vi "Settings Dialog.vi"(8 "error in (no error)":errorcluster, 11 "Settings in":T1={"Hardware Configuration"={"DAQmx Channel"="", "Sample Rate"=1000.0, "DAQmx Task"="", "ResetInterp"=FALSE, "GainConstants"=[], "FilterCoefficients"=[], "ChannelNames"=[], "ActiveChannels"=[], "Display Rate"=1000, "ResponseExtension"=TRUE}, "Logging Configuration"={"Log File Base Path"=path "", "Samples to Save"=0, "Trigger - Threshold"=0.0, "Trigger - Channel"=0, "Always Log"=FALSE, "External Trigger"=FALSE, "External Trigger Armed"=FALSE, "TDMS File Reference"=refnum, "DAQVersion"="", "SWVersion"="", "CircSamples"=0, "BeepWhenComplete"=FALSE, "ChannelConfig"=[], "ActiveChannels"=[], "Title"="", "Description"="", "ChannelNames"=[], "ResponseExtension"=TRUE}}) -> (0 "error out":errorcluster, 1 "Cancelled?":bool=TRUE, 2 "UI Refresh Needed?":bool, 3 "Settings out":T1={"Hardware Configuration"={"DAQmx Channel"="", "Sample Rate"=1000.0, "DAQmx Task"="", "ResetInterp"=FALSE, "GainConstants"=[], "FilterCoefficients"=[], "ChannelNames"=[], "ActiveChannels"=[], "Display Rate"=1000, "ResponseExtension"=TRUE}, "Logging Configuration"={"Log File Base Path"=path "C:/Users/jpassiak/Documents/LabVIEW Data/Logged Data.tdms", "Samples to Save"=0, "Trigger - Threshold"=0.0, "Trigger - Channel"=0, "Always Log"=FALSE, "External Trigger"=FALSE, "External Trigger Armed"=FALSE, "TDMS File Reference"=refnum, "DAQVersion"="", "SWVersion"="", "CircSamples"=0, "BeepWhenComplete"=FALSE, "ChannelConfig"=[], "ActiveChannels"=[], "Title"="", "Description"="", "ChannelNames"=[], "ResponseExtension"=TRUE}})   [LabVIEW 2017, in "Settings.lvlib"]
doc: "Dialog for selecting user specified settings."
uses:
  Settings.lvlib
  Settings.ctl
  Acquisition/Hardware Configuration.ctl
  Logging/Logging Configuration.ctl
  <vilib>/Utility/xml.llb/Write to XML File(string).vi
  Acquisition/Acquisition.lvlib
  Logging/Logging.lvlib
panel:
  in  "Tab Control 2":enum32{"Logging", "Channels", "Description"}(tab)=enum."Description"
  in  "Log File Path":path
  in  "Always Log":bool
  in  "Trigger Threshold\n [mm/s]":dbl min=0.0 max=100.0
  in  "Trigger Channel":u32(ring)=1 items=["CH1X", "CH1Y", "CH1Z"]
  in  "Channel Trigger":bool
  in  "Record Length [s]":u32=2
  in  "External Trigger":bool
  in  "Sample Rate [Hz]":u32=1000 min=4 max=1000
  in  "Pre-Trigger Buffer[s]":u32=2
  in  "Beep When Complete":bool=TRUE
  in  "Sensor response extension to 1Hz":bool=TRUE
  in  "Display Rate":i32=250 min=250 max=1000 step=10
  in  "Multicolumn Listbox":i32[](listbox)
  in  "Select Channels":i32[](listbox)
  in  "Description":string="..."
  in  "Title":string="Vibration Measurement"
  in  "Cancel Button":bool
  in  "OK Button":bool
  # "Non visible portion of dialog (needed for connector pane)."
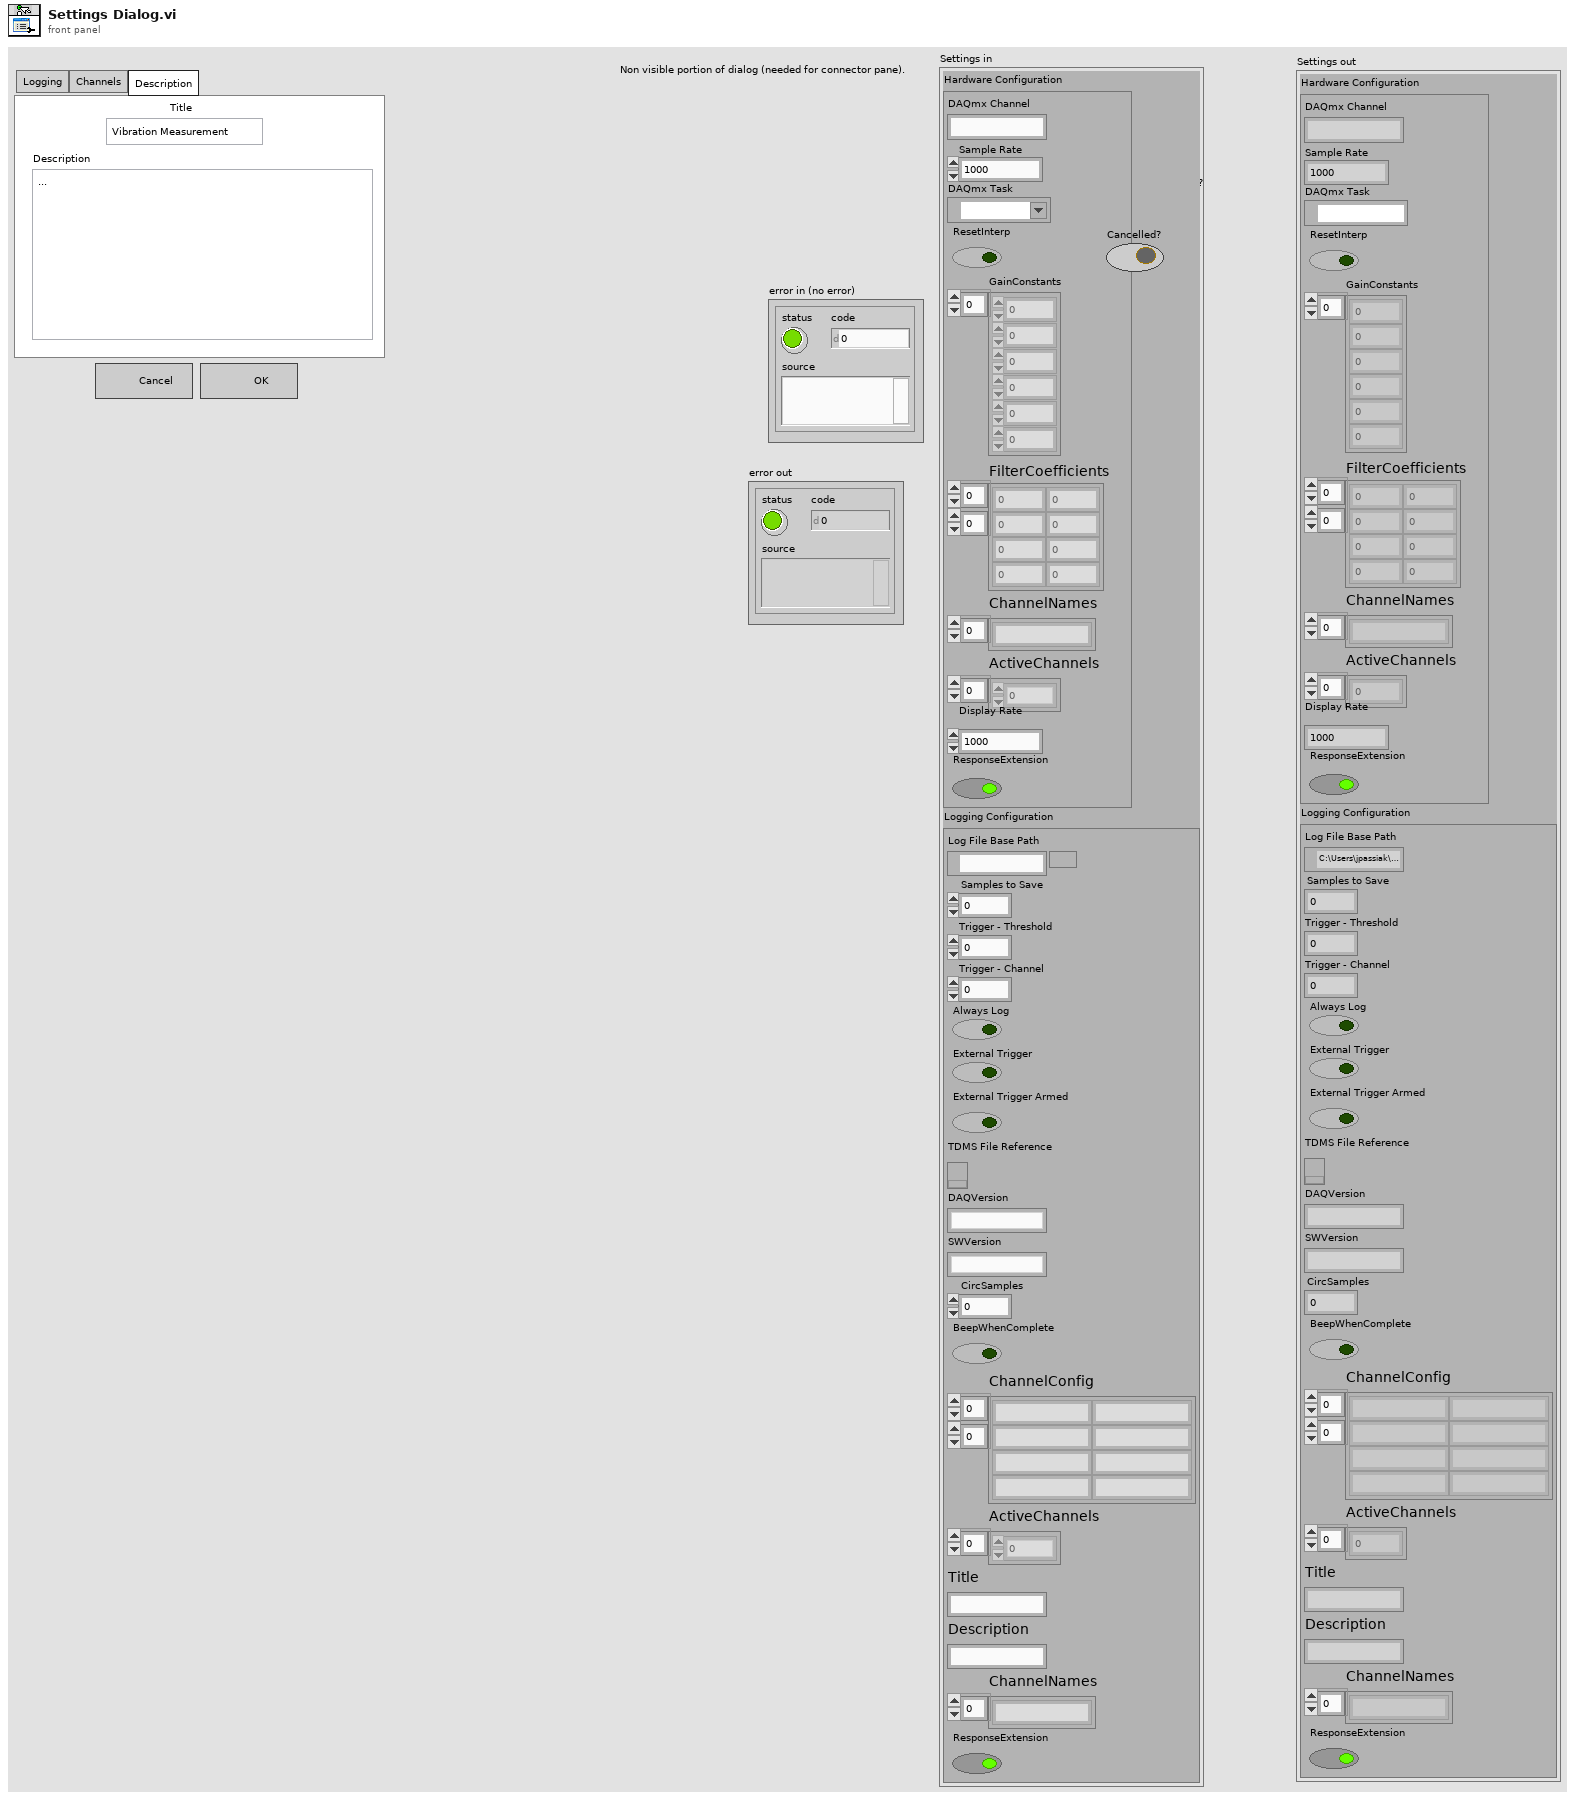
[diagram p1: front panel]
types:
  T1 = typedef "Settings.lvlib/Settings.ctl" = cluster{"Hardware Configuration":T2, "Logging Configuration":T3}
  T2 = typedef "Acquisition.lvlib/Hardware Configuration.ctl" = cluster{"DAQmx Channel":string, "Sample Rate":dbl, "DAQmx Task":refnum<k21>, "ResetInterp":bool, "GainConstants":dbl[], "FilterCoefficients":dbl[][], "ChannelNames":string[], "ActiveChannels":i32[], "Display Rate":i32, "ResponseExtension":bool}
  T3 = typedef "Logging.lvlib/Logging Configuration.ctl" = cluster{"Log File Base Path":path, "Samples to Save":u32, "Trigger - Threshold":dbl, "Trigger - Channel":u32, "Always Log":bool, "External Trigger":bool, "External Trigger Armed":bool, "TDMS File Reference":refnum<k34>, "DAQVersion":string, "SWVersion":string, "CircSamples":u32, "BeepWhenComplete":bool, "ChannelConfig":string[][], "ActiveChannels":i32[], "Title":string, "Description":string, "ChannelNames":string[], "ResponseExtension":bool}
  T4 = typedef "LVPoint32TypeDef.ctl" = cluster{"Horizontal":i32, "Vertical":i32}
  T5 = typedef "LVRowAndColumnTypeDef.ctl" = cluster{"Row":i32, "Column":i32}
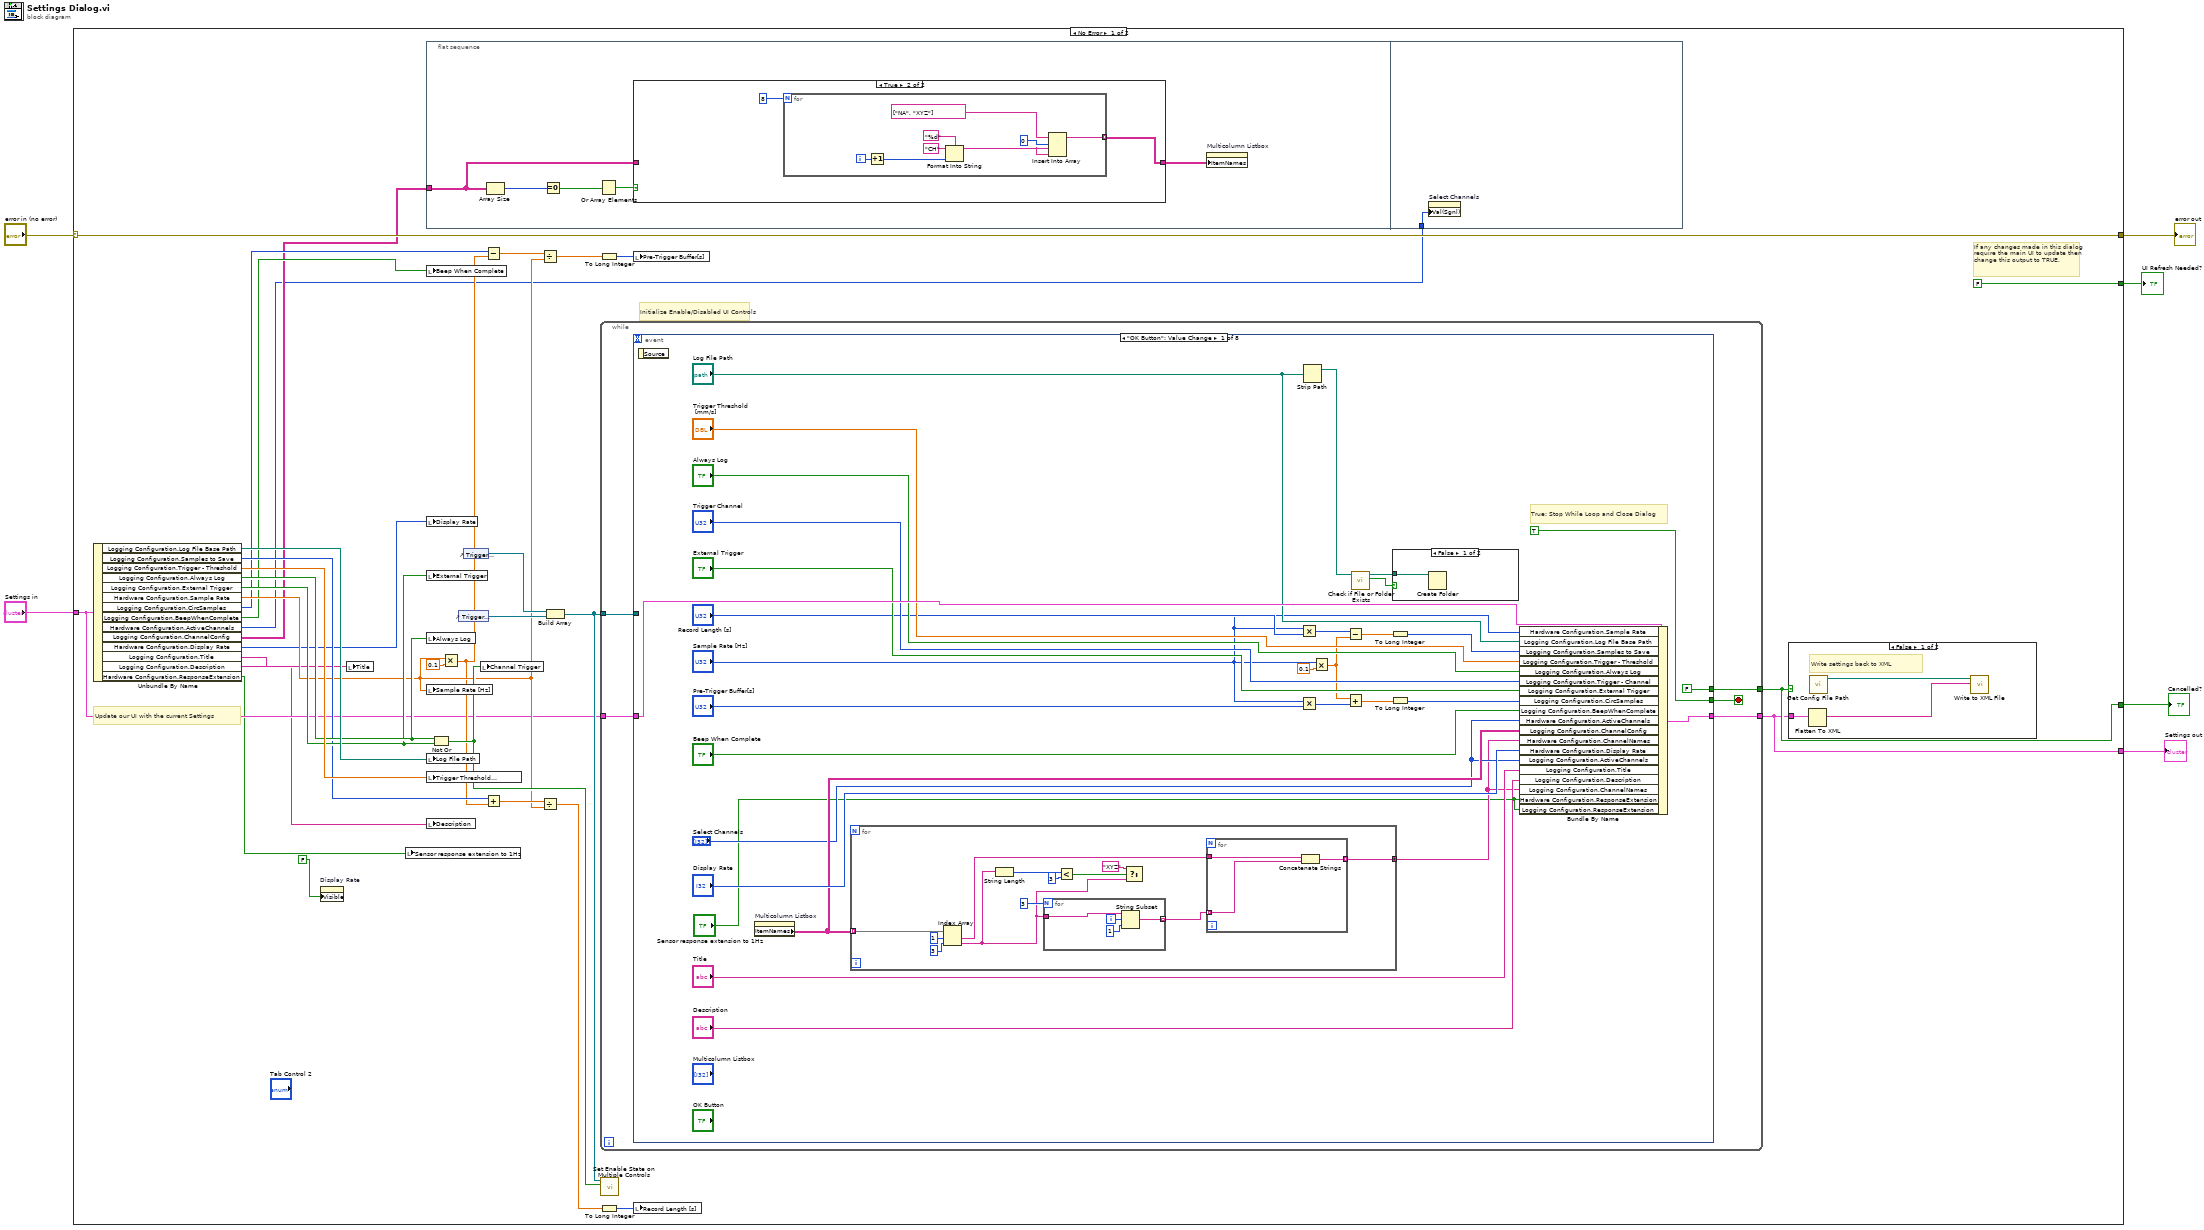
[diagram p0: block diagram]
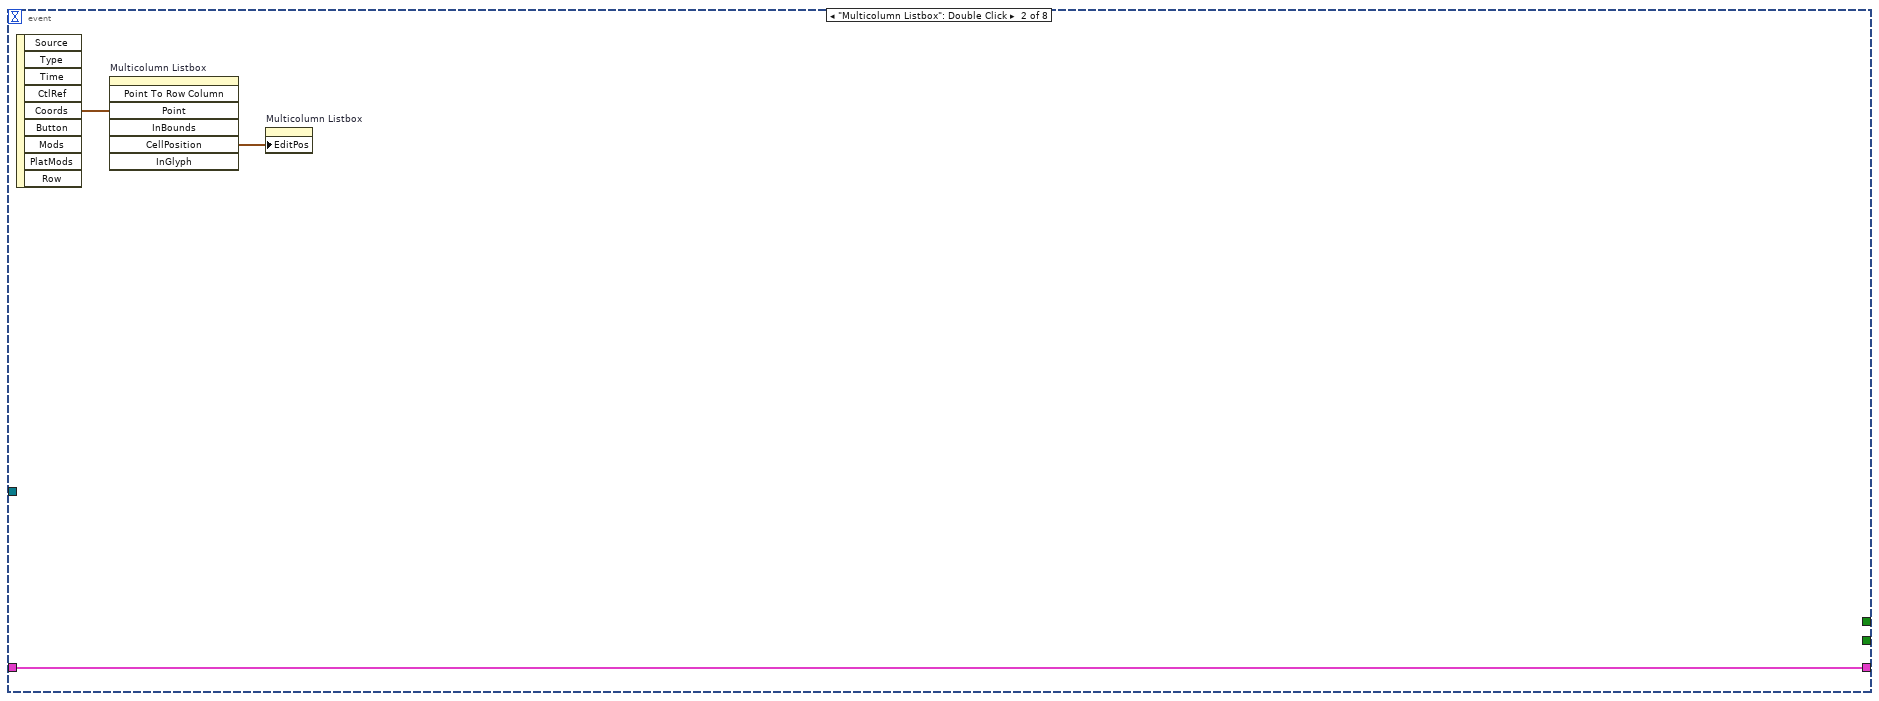
[diagram p4: hidden frame]
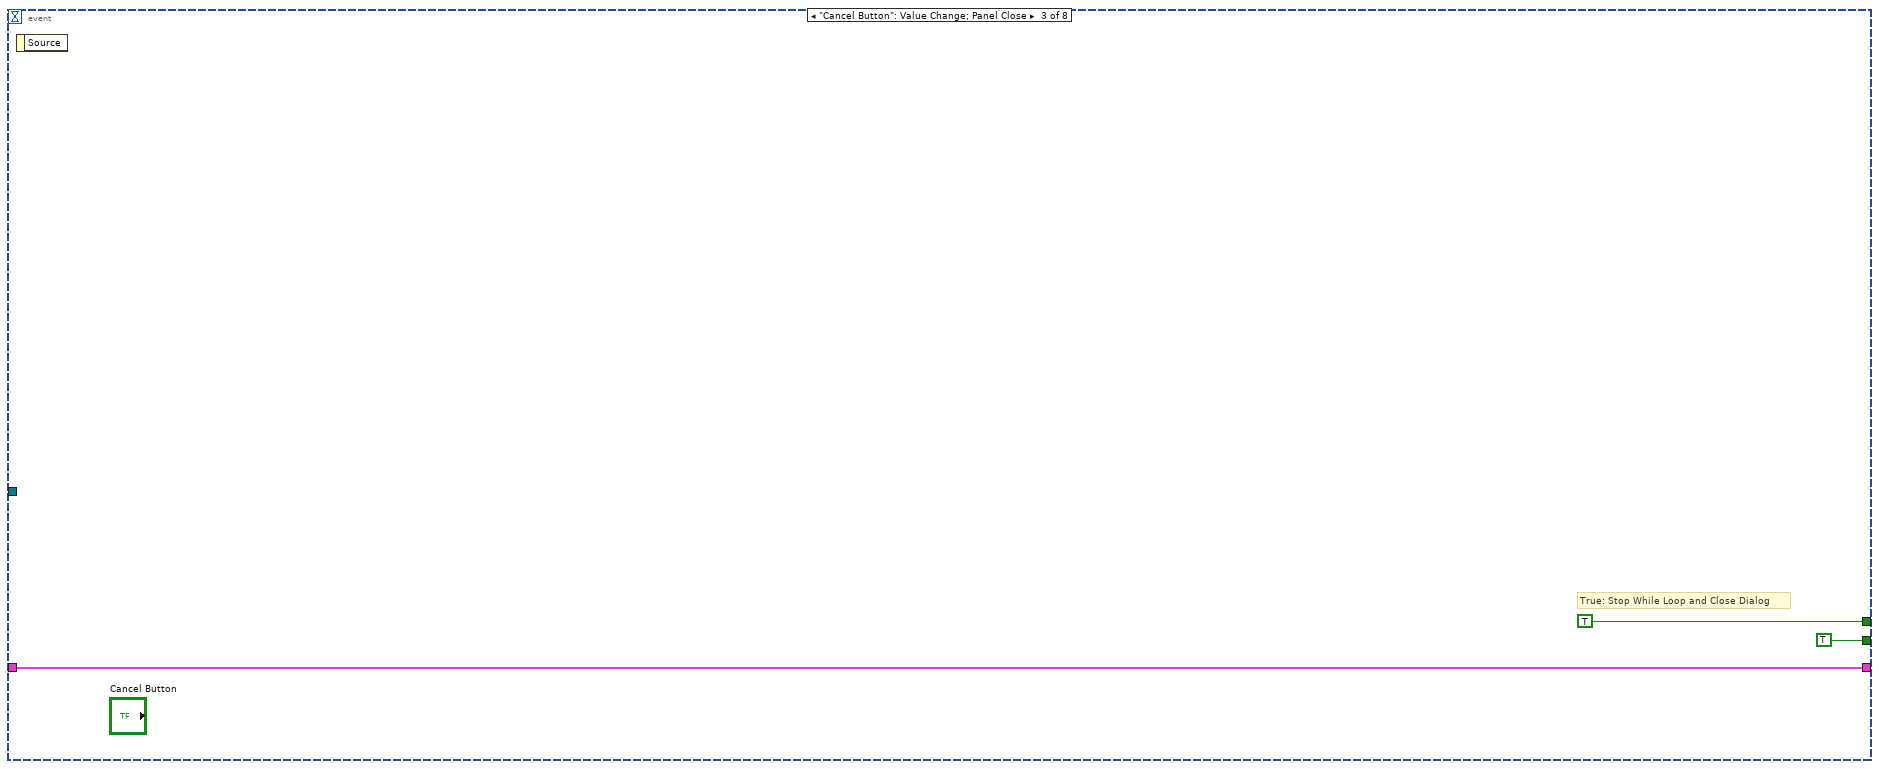
[diagram p5: hidden frame]
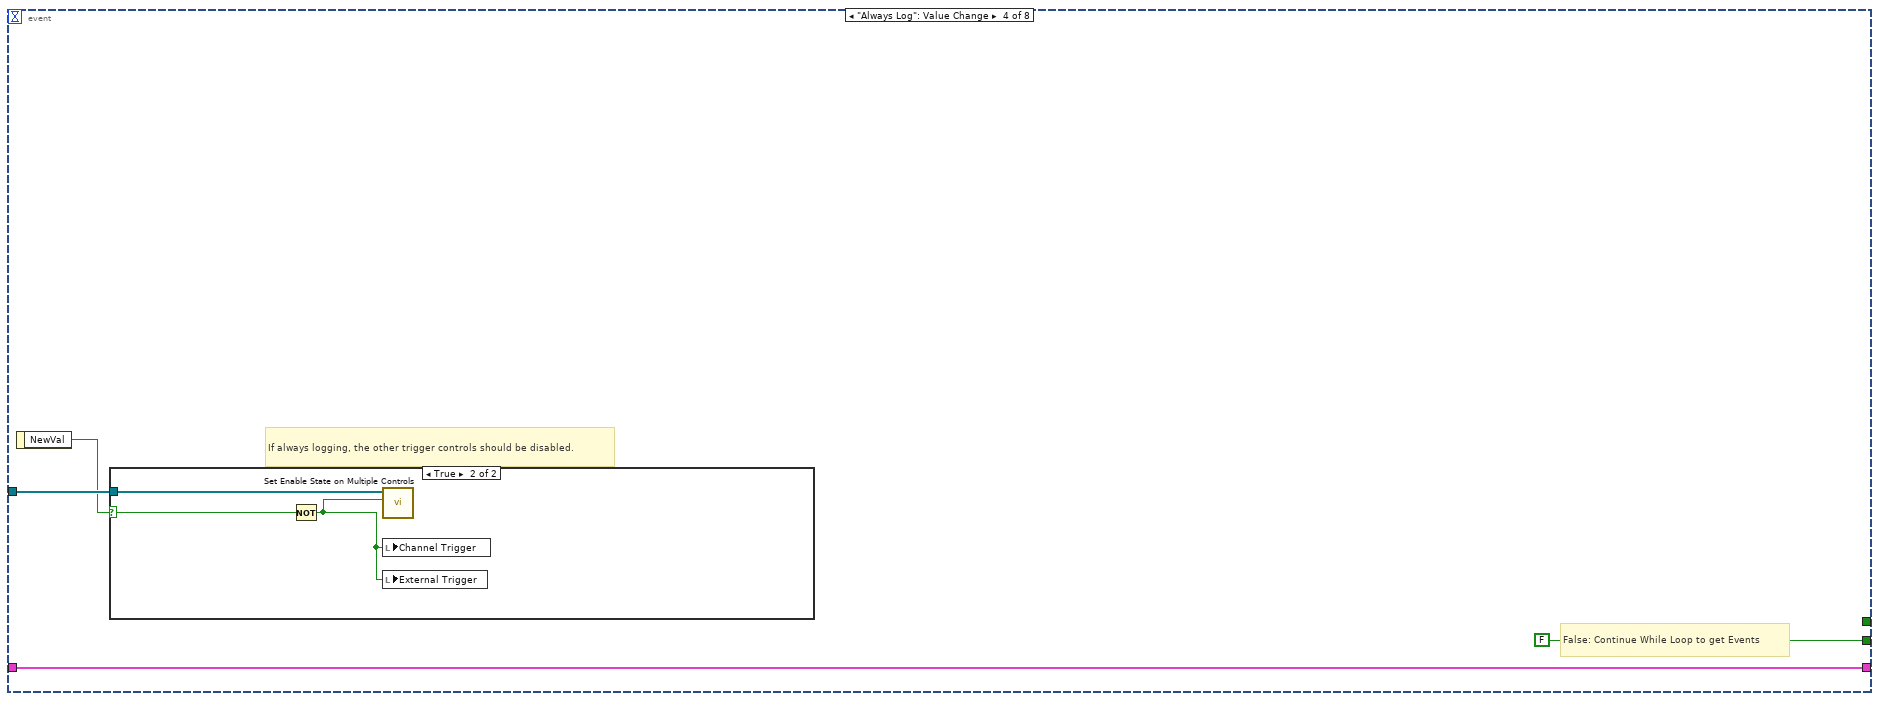
[diagram p6: hidden frame]
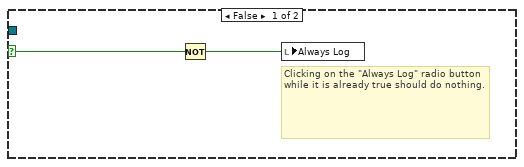
[diagram p7: hidden frame]
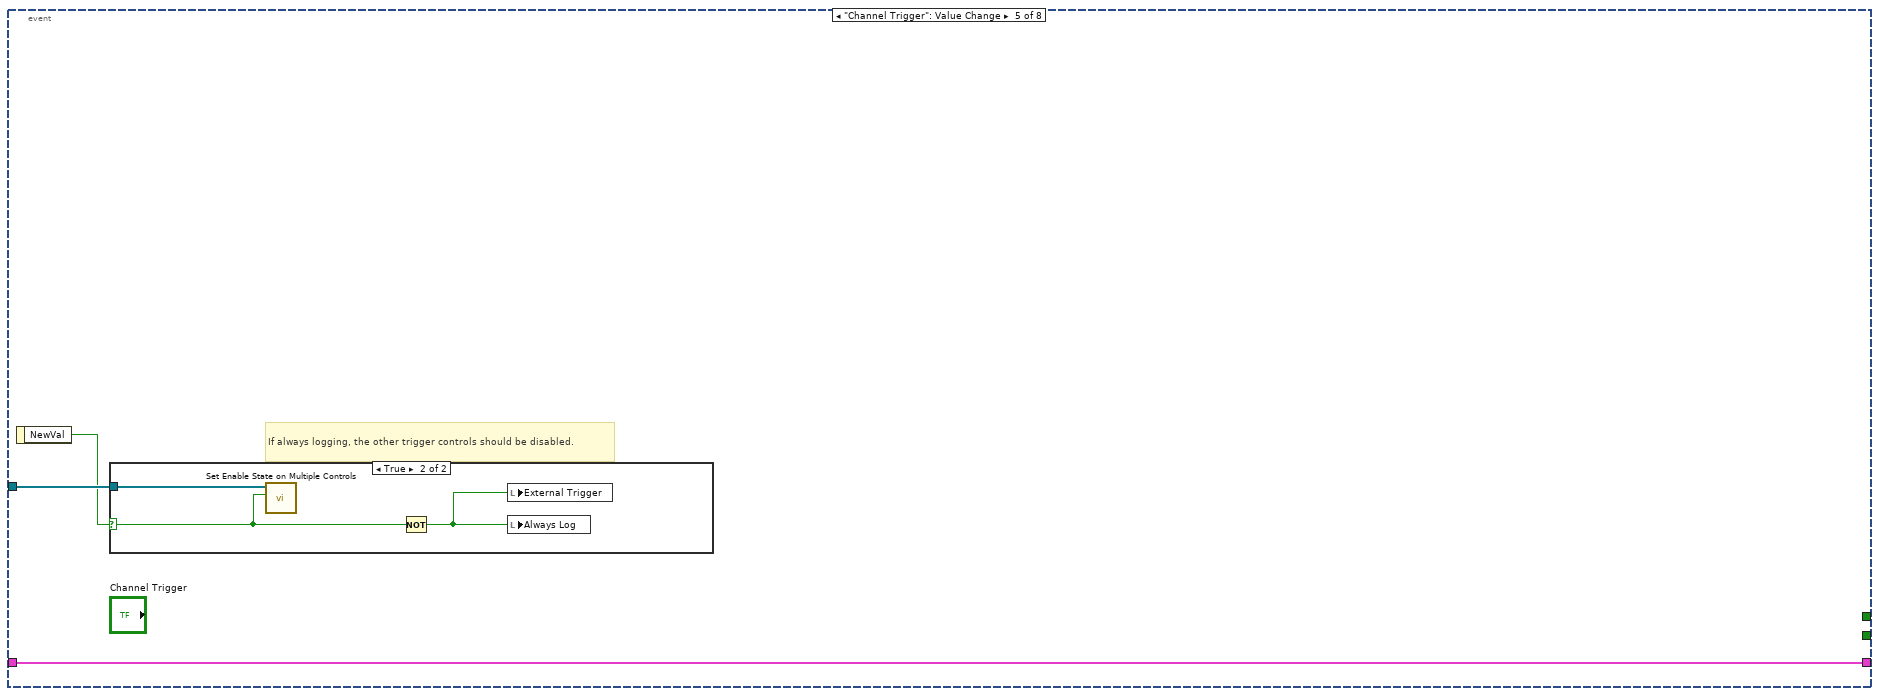
[diagram p8: hidden frame]
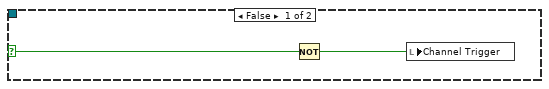
[diagram p9: hidden frame]
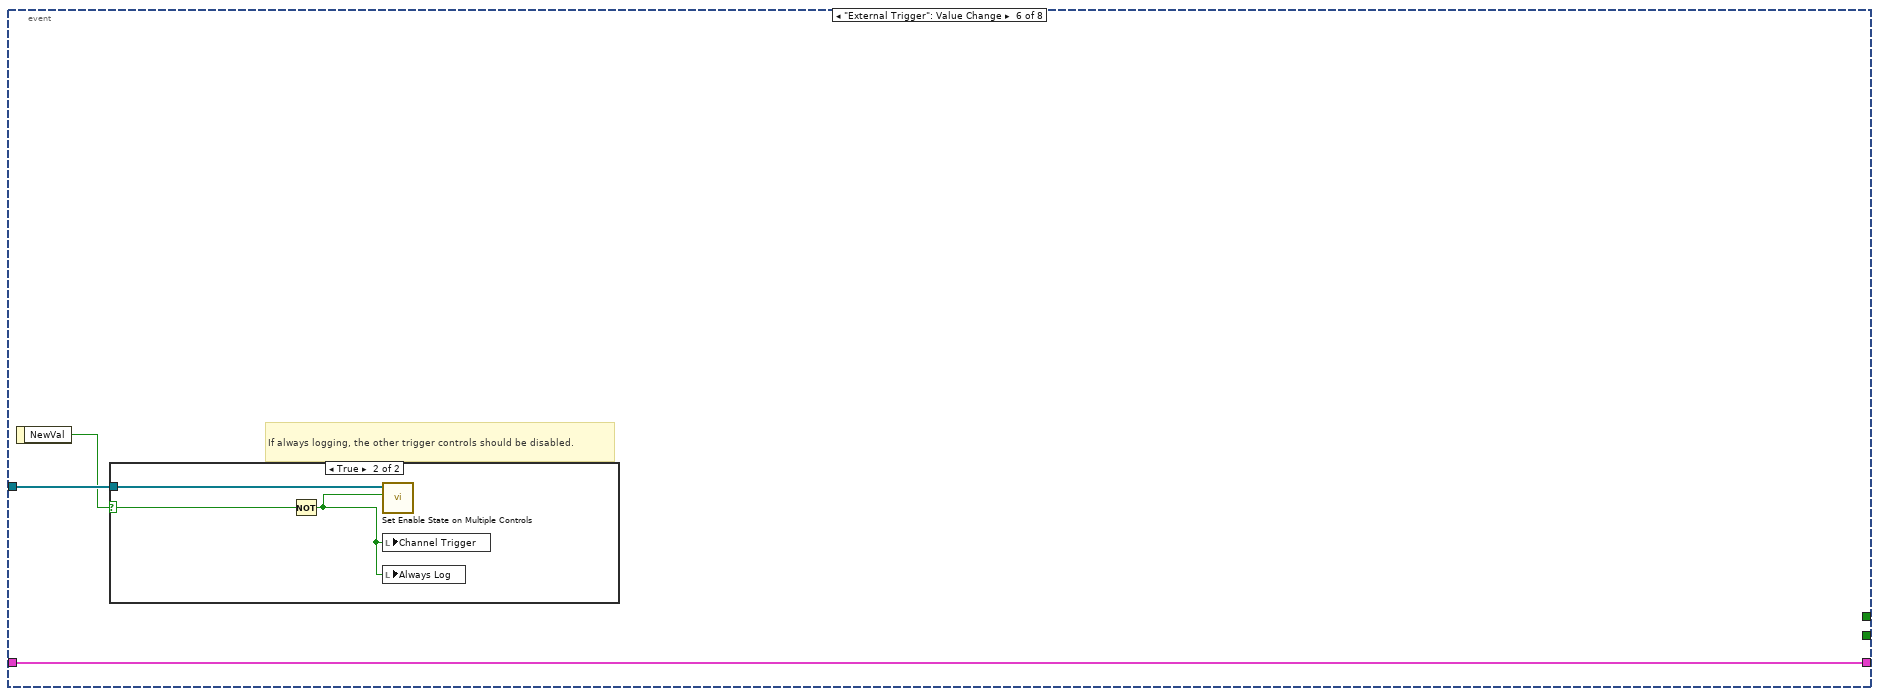
[diagram p10: hidden frame]
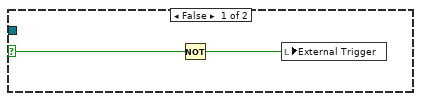
[diagram p11: hidden frame]
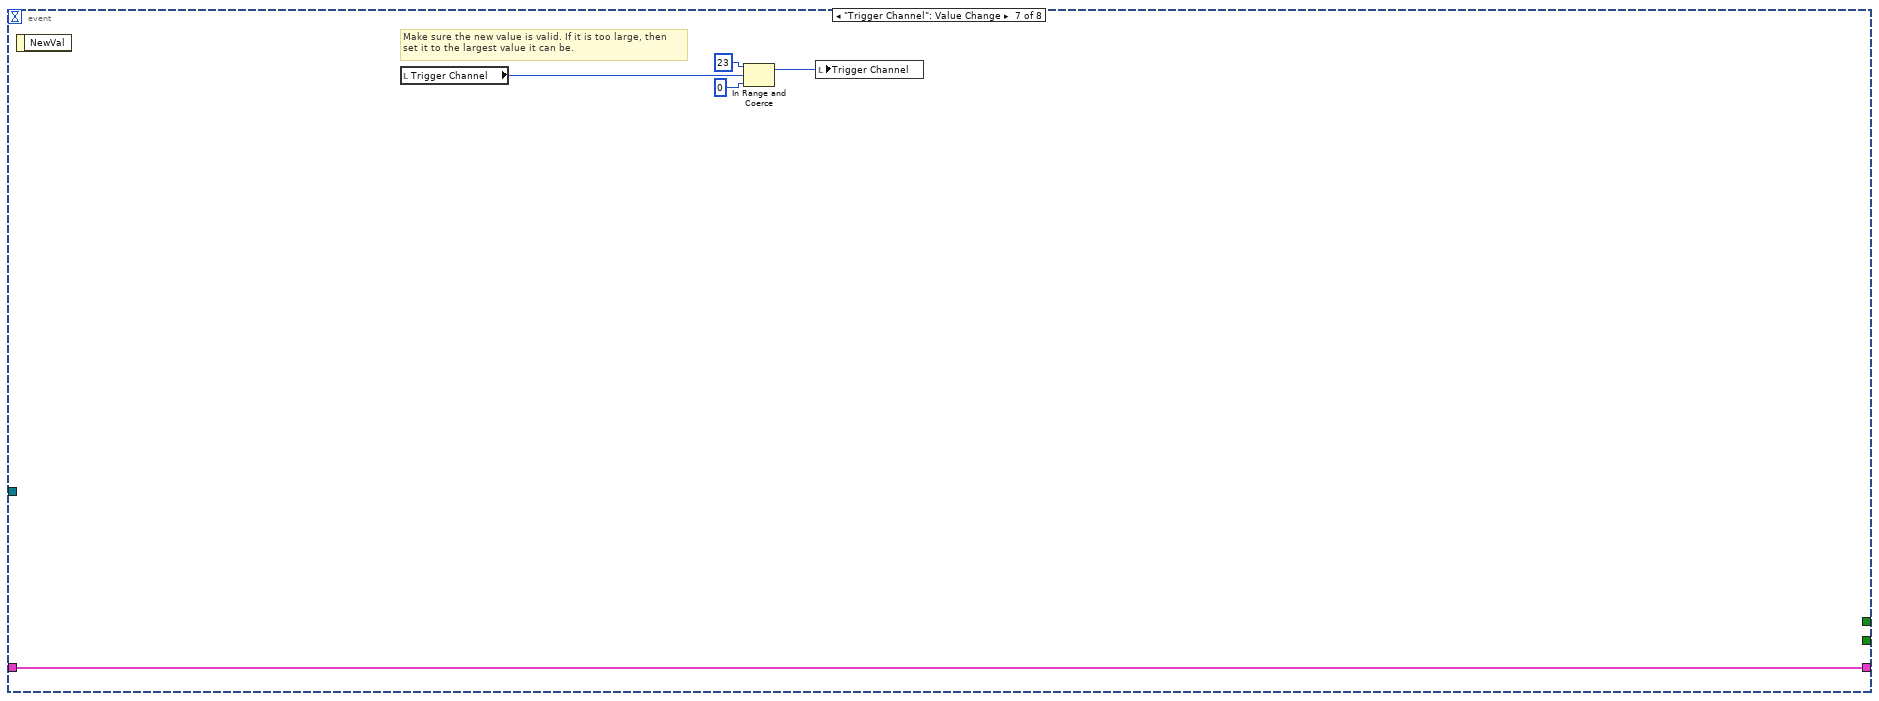
[diagram p12: hidden frame]
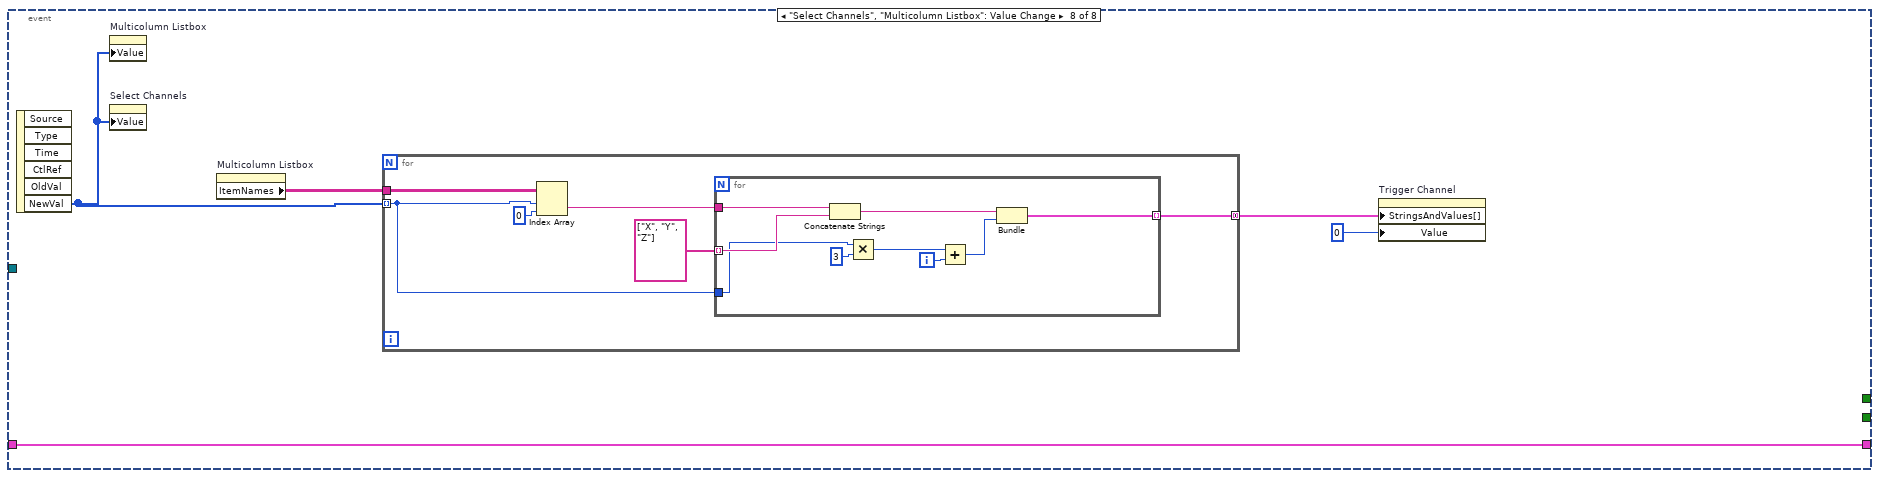
[diagram p13: hidden frame]
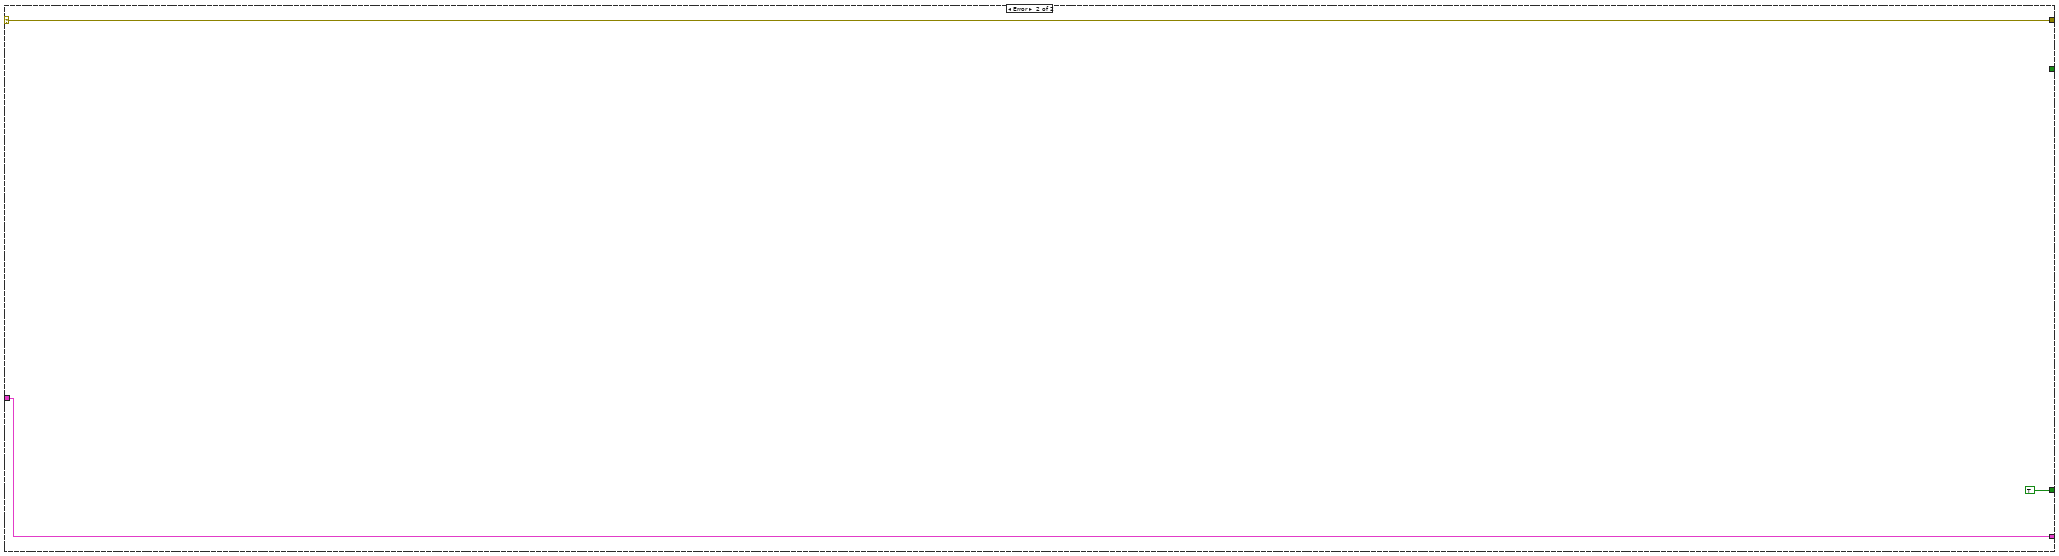
[diagram p15: hidden frame]
diagram:
  n1 = case shown="No Error" "error in (no error)" {
    selector: "error in (no error)" -> [w38 w173]
    tunnel: [w38 w173] -> w6
    tunnel: "Settings in" -> [w11 w172]
    tunnel: [w35 w172] -> w4
    tunnel: [FALSE ("UI Refresh Needed?") _] -> w3
    tunnel: [w36 TRUE ("UI Refresh Needed?")] -> w2
    frame No Error {
      # "Update our UI with the current Settings"
      # "Initialize Enable/Disabled UI Controls"
      # "If any changes made in this dialog require the main UI to update then change this output to TRUE."
      n2 = Unbundle By Name(w11) -> ("Logging Configuration.Log File Base Path"=w34:path, "Logging Configuration.Samples to Save"=w21:u32, "Logging Configuration.Trigger - Threshold"=w33:dbl, "Logging Configuration.Always Log"=w24:bool, "Logging Configuration.External Trigger"=w23:bool, "Hardware Configuration.Sample Rate"=w19:dbl, "Logging Configuration.CircSamples"=w17:u32, "Logging Configuration.BeepWhenComplete"=w15:bool, "Hardware Configuration.ActiveChannels"=w12:i32[], "Logging Configuration.ChannelConfig"=w13:string[][], "Hardware Configuration.Display Rate"=w14:i32, "Logging Configuration.Title"=w10:string, "Logging Configuration.Description"=w9:string, "Hardware Configuration.ResponseExtension"=w7:bool)
      n3 = property on="Display Rate" class="DigNum (strict)"("Visible"=FALSE) -> ()  [unwired: 2 in, 2 out]
      n4 = local write "Title"(w10) -> ()
      n5 = local write "Sensor response extension to 1Hz"(w7) -> ()
      n6 = flat-sequence {
        tunnel: w13 -> [w40]
        tunnel: w12 -> [w55]
        frame #0 {
          n7 = Array Size(array=w40) -> (size(s)=w41:i32[])
          n8 = Equal To 0?(x=w41) -> (x = 0?=w42:bool[])
          n9 = Or Array Elements(Boolean array=w42) -> (logical OR=w39:bool)
          n10 = case shown="True" w39 {
            tunnel: w40 -> [w44 _]
            tunnel: [w44 w45] -> w43
            frame False {
            }
            frame True {
              n11 = for {
                N: 8 -> [_]
                tunnel: [w49] -> w45 mode=indexing
                i -> [w52]
                n12 = Increment(x=w52) -> (x+1=w47:i32)
                n13 = Format Into String(format string="%d", initial string="CH", w47) -> (resulting string=w48:string)  [unwired: 1 in, 1 out]
                n14 = Insert Into Array(array=string[] ["NA", "XYZ"], index=0, new element #1=w48, new element #2=w48) -> (w49:string[])
              }
            }
          }
          n15 = property on="Multicolumn Listbox" class="MCListbox (strict)"("ItemNames"=w43) -> ()  [unwired: 2 in, 2 out]
        }
        frame #1 {
          n16 = property on="Select Channels" class="LstBox (strict)"("Val(Sgnl)"=w55) -> ()  [unwired: 2 in, 2 out]
        }
      }
      n17 = local write "Beep When Complete"(w15) -> ()
      n18 = local write "Display Rate"(w14) -> ()
      n19 = local write "External Trigger"(w23) -> ()
      n20 = local write "Always Log"(w24) -> ()
      n21 = local write "Sample Rate [Hz]"(w19) -> ()
      n22 = local write "Log File Path"(w34) -> ()
      n23 = local write "Trigger Threshold\n [mm/s]"(w33) -> ()
      n24 = local write "Description"(w9) -> ()
      n25 = Not Or(1:w23, 2:w24) -> (0:w30:bool)
      n26 = Multiply(x=w19, y=0.1) -> (x*y=w18:dbl)
      n27 = control-ref of="Trigger Threshold\n [mm/s]"() -> (w29:refnum<vi>)
      n28 = control-ref of="Trigger Channel"() -> (w31:refnum<vi>)
      n29 = local write "Channel Trigger"(w30) -> ()
      n30 = Subtract(x=w17, y=w18) -> (x-y=w16:dbl)
      n31 = Add(x=w21, y=w18) -> (x+y=w22:dbl)
      n32 = Divide(x=w16, y=w19) -> (x/y=w28:dbl)
      n33 = Divide(x=w22, y=w19) -> (x/y=w25:dbl)
      n34 = Build Array(w31, w29) -> (w32:refnum<vi>[])
      n35 = To Long Integer(number=w28) -> (32bit integer=w27:i32)
      n36 = To Long Integer(number=w25) -> (32bit integer=w26:i32)
      n37 = while {
        tunnel: [w60] -> w36
        tunnel: [w59] -> w35
        tunnel: w11 -> [w58]
        tunnel: w32 -> [w56]
        stop <- w57 stop-if-true
        n38 = event shown="[0] \"OK Button\": Value Change" {
          selector: _ -> [_ _ _ _ _ _ _ _]
          dyn-events: _ -> [_ _ _ _ _ _ _ _]
          timeout: _ -> [_ _ _ _ _ _ _ _]
          tunnel: [w89 w114 w117 w121 w129 w137 w144 w152] -> w59
          tunnel: w58 -> [w88 w114 w117 w121 w129 w137 w144 w152]
          tunnel: [FALSE ("UI Refresh Needed?") _ TRUE ("UI Refresh Needed?") _ _ _ _ _] -> w60
          tunnel: [TRUE _ TRUE FALSE _ _ _ _] -> w57
          tunnel: w56 -> [_ _ _ w119 w128 w136 _ _]
          event "OK Button": Value Change {
            # "True: Stop While Loop and Close Dialog"
            n39 = event-data() -> ()  [unwired: 1 in, 1 out]
            n40 = property on="Multicolumn Listbox" class="MCListbox (strict)"() -> ("ItemNames"=w66:string[][])  [unwired: 2 in, 2 out]
            n41 = for {
              tunnel: w66 -> [w103] mode=indexing
              tunnel: [w101] -> w62 mode=concatenating
              n42 = Index Array(array=w103, index #1=1 ("disabled index (col)"), index #2=3 ("index")) -> (element #1=w102:string, element #2=w93:string)
              n43 = String Length(string=w93) -> (length=w96:i32)
              n44 = for {
                N: 3 -> [_]
                tunnel: w93 -> [w105]
                tunnel: [w104] -> w98 mode=indexing
                i -> [w106]
                n45 = String Subset(string=w105, offset (0)=w106, length (rest)=1 ("length (rest)")) -> (substring=w104:string)
              }
              n46 = Less?(x=w96, y=3) -> (x < y?=w94:bool)
              n47 = Select(t="XYZ", s=w94, f=w93) -> ()  [unwired: 1 out]
              n48 = for {
                tunnel: w102 -> [w110]
                tunnel: w98 -> [w109] mode=indexing
                tunnel: [w108] -> w101 mode=indexing
                n49 = Concatenate Strings(w110, w109) -> (w108:string)
              }
            }
            n50 = Multiply(x="Sample Rate [Hz]", y="Record Length [s]") -> (x*y=w77:u32)
            n51 = Multiply(x="Sample Rate [Hz]", y="Pre-Trigger Buffer[s]") -> (x*y=w70:u32)
            n52 = Strip Path(path="Log File Path") -> (stripped path=w82:path)  [unwired: 1 out]
            n53 = Multiply(x="Sample Rate [Hz]", y=0.1) -> (x*y=w69:dbl)
            n54 = Subtract(x=w77, y=w69) -> (x-y=w73:dbl)
            n55 = Add(x=w69, y=w70) -> (x+y=w72:dbl)
            n56 = call <vilib>:"Check if File or Folder Exists.vi"("path"=w82) -> ("file or folder exists?"=w80:bool, "dup path"=w79:path)  [unwired: 8 in, 1 out]
            n57 = To Long Integer(number=w73) -> (32bit integer=w74:i32)
            n58 = To Long Integer(number=w72) -> (32bit integer=w71:i32)
            n59 = case shown="False" w80 {
              tunnel: w79 -> [w111 _]
              frame False {
                n60 = Create Folder(path (use dialog)=w111) -> ()  [unwired: 2 in, 3 out]
              }
              frame True {
              }
            }
            n61 = Bundle By Name(cluster=w88, "Hardware Configuration.Sample Rate"="Sample Rate [Hz]", "Logging Configuration.Log File Base Path"="Log File Path", "Logging Configuration.Samples to Save"=w74, "Logging Configuration.Trigger - Threshold"="Trigger Threshold\n [mm/s]", "Logging Configuration.Always Log"="Always Log", "Logging Configuration.Trigger - Channel"="Trigger Channel", "Logging Configuration.External Trigger"="External Trigger", "Logging Configuration.CircSamples"=w71, "Logging Configuration.BeepWhenComplete"="Beep When Complete", "Hardware Configuration.ActiveChannels"="Select Channels", "Logging Configuration.ChannelConfig"=w66, "Hardware Configuration.ChannelNames"=w62, "Hardware Configuration.Display Rate"="Display Rate", "Logging Configuration.ActiveChannels"="Select Channels", "Logging Configuration.Title"="Title", "Logging Configuration.Description"="Description", "Logging Configuration.ChannelNames"=w62, "Hardware Configuration.ResponseExtension"="Sensor response extension to 1Hz", "Logging Configuration.ResponseExtension"="Sensor response extension to 1Hz") -> (w89:T1)
          }
          event "Multicolumn Listbox": Double Click {
            n62 = event-data() -> ("Coords"=w113:T4)  [unwired: 1 in, 8 out]
            n63 = invoke on="Multicolumn Listbox" class="MCListbox (strict)" method="Point To Row Column"("Point"=w113) -> ("CellPosition"=w112:T5)  [unwired: 6 in, 6 out]
            n64 = property on="Multicolumn Listbox" class="MCListbox (strict)"("EditPos"=w112) -> ()  [unwired: 2 in, 2 out]
          }
          event "Cancel Button": Value Change; Panel Close {
            # "True: Stop While Loop and Close Dialog"
            n65 = event-data() -> ()  [unwired: 1 in, 1 out]
          }
          event "Always Log": Value Change {
            # "False: Continue While Loop to get Events"
            # "If always logging, the other trigger controls should be disabled."
            n66 = event-data() -> ("NewVal"=w118:bool)  [unwired: 1 in]
            n67 = case shown="True" w118 {
              selector: w118 -> [w123 w126]
              tunnel: w119 -> [_ w125]
              frame False {
                # "Clicking on the \"Always Log\" radio button while it is already true should do nothing."
                n68 = Not(x=w123) -> (.not. x?=w122:bool)
                n69 = local write "Always Log"(w122) -> ()
              }
              frame True {
                n70 = Not(x=w126) -> (.not. x?=w124:bool)
                n71 = call "Set Enable State on Multiple Controls.vi"("Enable?"=w124, "Controls"=w125) -> ()  [unwired: 10 in]
                n72 = local write "Channel Trigger"(w124) -> ()
                n73 = local write "External Trigger"(w124) -> ()
              }
            }
          }
          event "Channel Trigger": Value Change {
            # "If always logging, the other trigger controls should be disabled."
            n74 = event-data() -> ("NewVal"=w127:bool)  [unwired: 1 in]
            n75 = case shown="True" w127 {
              selector: w127 -> [w131 w133]
              tunnel: w128 -> [_ w134]
              frame False {
                n76 = Not(x=w131) -> (.not. x?=w130:bool)
                n77 = local write "Channel Trigger"(w130) -> ()
              }
              frame True {
                n78 = call "Set Enable State on Multiple Controls.vi"("Enable?"=w133, "Controls"=w134) -> ()  [unwired: 10 in]
                n79 = Not(x=w133) -> (.not. x?=w132:bool)
                n80 = local write "External Trigger"(w132) -> ()
                n81 = local write "Always Log"(w132) -> ()
              }
            }
          }
          event "External Trigger": Value Change {
            # "If always logging, the other trigger controls should be disabled."
            n82 = event-data() -> ("NewVal"=w135:bool)  [unwired: 1 in]
            n83 = case shown="True" w135 {
              selector: w135 -> [w139 w141]
              tunnel: w136 -> [_ w142]
              frame False {
                n84 = Not(x=w139) -> (.not. x?=w138:bool)
                n85 = local write "External Trigger"(w138) -> ()
              }
              frame True {
                n86 = Not(x=w141) -> (.not. x?=w140:bool)
                n87 = call "Set Enable State on Multiple Controls.vi"("Enable?"=w140, "Controls"=w142) -> ()  [unwired: 10 in]
                n88 = local write "Channel Trigger"(w140) -> ()
                n89 = local write "Always Log"(w140) -> ()
              }
            }
          }
          event "Trigger Channel": Value Change {
            # "Make sure the new value is valid. If it is too large, then\nset it to the largest value it can be."
            n90 = event-data() -> ()  [unwired: 1 in, 1 out]
            n91 = local read "Trigger Channel"() -> (w145:u32)
            n92 = In Range and Coerce(upper limit=u32 23, x=w145, lower limit=u32 0) -> (coerced(x)=w146:u32)  [unwired: 1 out]
            n93 = local write "Trigger Channel"(w146) -> ()
          }
          event "Select Channels", "Multicolumn Listbox": Value Change {
            n94 = event-data() -> ("NewVal"=w151:i32[])  [unwired: 1 in, 5 out]
            n95 = property on="Multicolumn Listbox" class="MCListbox (strict)"("Value"=w151) -> ()  [unwired: 2 in, 2 out]
            n96 = property on="Select Channels" class="LstBox (strict)"("Value"=w151) -> ()  [unwired: 2 in, 2 out]
            n97 = property on="Multicolumn Listbox" class="MCListbox (strict)"() -> ("ItemNames"=w150:string[][])  [unwired: 2 in, 2 out]
            n98 = for {
              tunnel: w151 -> [w155] mode=indexing
              tunnel: w150 -> [w158]
              tunnel: [w153] -> w149 mode=concatenating
              n99 = Index Array(array=w158, index (row)=w155, index (col)=0 ("disabled index (col)")) -> (element=w156:string)
              n100 = for {
                tunnel: w156 -> [w167]
                tunnel: w155 -> [w164]
                tunnel: string[] ["X", "Y", "Z"] -> [w166] mode=indexing
                tunnel: [w165] -> w153 mode=indexing
                i -> [w160]
                n101 = Concatenate Strings(w167, w166) -> (w159:string)
                n102 = Multiply(x=w164, y=3) -> (x*y=w161:i32)
                n103 = Add(x=w161, y=w160) -> (x+y=w162:i32)
                n104 = Bundle(w159, w162) -> (w165:cluster{string, i32})  [unwired: 1 in]
              }
            }
            n105 = property on="Trigger Channel" class="Ring (strict)"("StringsAndValues[]"=w149, "Value"=0) -> ()  [unwired: 2 in, 2 out]
          }
        }
      }
      n106 = call "Set Enable State on Multiple Controls.vi"("Enable?"=w30, "Controls"=w32) -> ()  [unwired: 10 in]
      n107 = local write "Pre-Trigger Buffer[s]"(w27) -> ()
      n108 = local write "Record Length [s]"(w26) -> ()
      n109 = case shown="False" w36 {
        tunnel: w35 -> [w169 _]
        frame False {
          # "Write settings back to XML"
          n110 = Flatten To XML(anything=w169) -> (xml string=w168:string)
          n111 = call "Get Config File Path.vi"() -> ("XML File Path"=w170:path)  [unwired: 10 in, 1 out]
          n112 = call-poly <vilib>:"Write to XML File.vi"("XML Input"=w168, "XML File Path"=w170) -> ()  [unwired: 7 in, 3 out]
        }
        frame True {
        }
      }
    }
    frame Error {
    }
  }
  "UI Refresh Needed?" <- w3
  "error out" <- w6
  "Settings out" <- w4
  "Cancelled?" <- w2
